vi "add two arrays using add numeric.vi"() -> ()   [LabVIEW 2010]
uses:
  <vilib>/Analysis/Matrix/NI_Matrix.lvlib
  <vilib>/Analysis/Matrix/Numeric/Add/Add - RM,RM.vi
  <vilib>/Analysis/Matrix/Datatypes/RealMatrix.ctl
panel:
  out "Real Matrix 3":T1
  in  "Real Matrix":T1
  in  "Real Matrix 2":T1
  in  "Cluster":T2
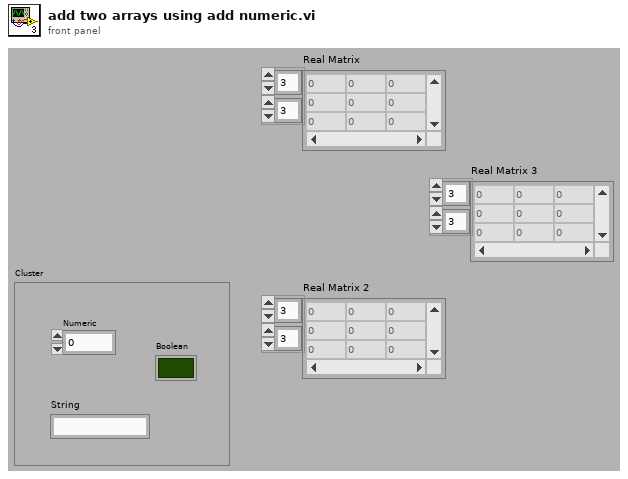
[diagram p1: front panel]
types:
  T1 = typedef "NI_Matrix.lvlib/RealMatrix.ctl" = dbl[][]
  T2 = cluster{"Numeric":dbl, "Boolean":bool, "String":string}
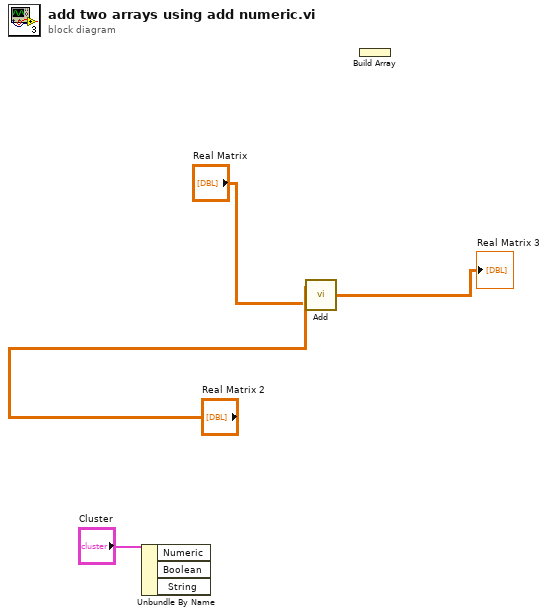
[diagram p0: block diagram]
diagram:
  n1 = Unbundle By Name("Cluster") -> ()  [unwired: 3 out]
  n2 = call-poly <vilib>:"Add.vi"("Real Matrix B"="Real Matrix", "Real Matrix A"="Real Matrix 2") -> ("A + B"=→"Real Matrix 3":T1)
  n3 = Build Array() -> ()  [unwired: 1 in, 1 out]
